vi "FL Convert fc to fs.vi"(8 "error in (no error)":errorcluster, 11 "old controller in":T1) -> (0 "error out":errorcluster, 3 "fuzzy system out":T2 {"user MF interpolating polynomials"."coa_x(y) coeff" format="%.4g"; "user MF interpolating polynomials"."Area(y) coeff" format="%.4g"; "user MF interpolating polynomials"."X(y) coeff" format="%.4g"; "user MF interpolating polynomials"."Y(x) coeff" format="%.4g"; "user MF interpolating polynomials"."Y" format="%.4g"; "user MF interpolating polynomials"."X" format="%.4g"; "defuzzification method" items=["Center of Area", "Modified Center of Area", "Center of Sums", "Center of Maximum", "Mean of Maximum"]; "rules"."consequents"."Var Index" min=0; "rules"."consequents"."Cond" items=["=", "!="]; "rules"."consequents"."MF Index" min=0; "rules"."antecedents"."Var Index" min=0; "rules"."antecedents"."Cond" items=["=", "!="]; "rules"."antecedents"."MF Index" min=0; "rules"."consequent implication" items=["Minimum", "Product"]; "rules"."antecedent connective" items=["AND (Minimum)", "AND (Product)", "OR (Maximum)", "OR (Probabilistic)"]; "output variables"."MFs"."shape" items=["Triangle", "Trapezoid", "Singleton", "Sigmoid", "Gaussian", "User-Defined"]; "input variables"."MFs"."shape" items=["Triangle", "Trapezoid", "Singleton", "Sigmoid", "Gaussian", "User-Defined"]})   [LabVIEW 2017, in "NI_Fuzzy_Logic_API.lvlib"]
uses:
  <vilib>/addons/Fuzzy Logic/NI_Fuzzy_Logic_API.lvlib
  <vilib>/addons/Fuzzy Logic/TypeDefs/FL System.ctl
  <vilib>/addons/Fuzzy Logic/TypeDefs/FL Variable.ctl
  <vilib>/addons/Fuzzy Logic/TypeDefs/FL Membership Function.ctl
  <vilib>/addons/Fuzzy Logic/TypeDefs/FL Membership Function Shape.ctl
  <vilib>/addons/Fuzzy Logic/TypeDefs/FL Rule.ctl
  <vilib>/addons/Fuzzy Logic/TypeDefs/FL Antecedent.ctl
  <vilib>/addons/Fuzzy Logic/TypeDefs/FL Modifier.ctl
  <vilib>/addons/Fuzzy Logic/TypeDefs/FL Antecedent Connective.ctl
  <vilib>/addons/Fuzzy Logic/TypeDefs/FL Consequent.ctl
  <vilib>/addons/Fuzzy Logic/TypeDefs/FL Consequent Implication.ctl
  <vilib>/addons/Fuzzy Logic/TypeDefs/FL Defuzzification.ctl
  <vilib>/addons/Fuzzy Logic/TypeDefs/FL Interpolating polynomials.ctl
  <vilib>/addons/Fuzzy Logic/Membership/FL Create Membership Function (Trapezoid).vi
  <vilib>/Analysis/NI_AALPro.lvlib
panel:
  # "IF"
  # "THEN"
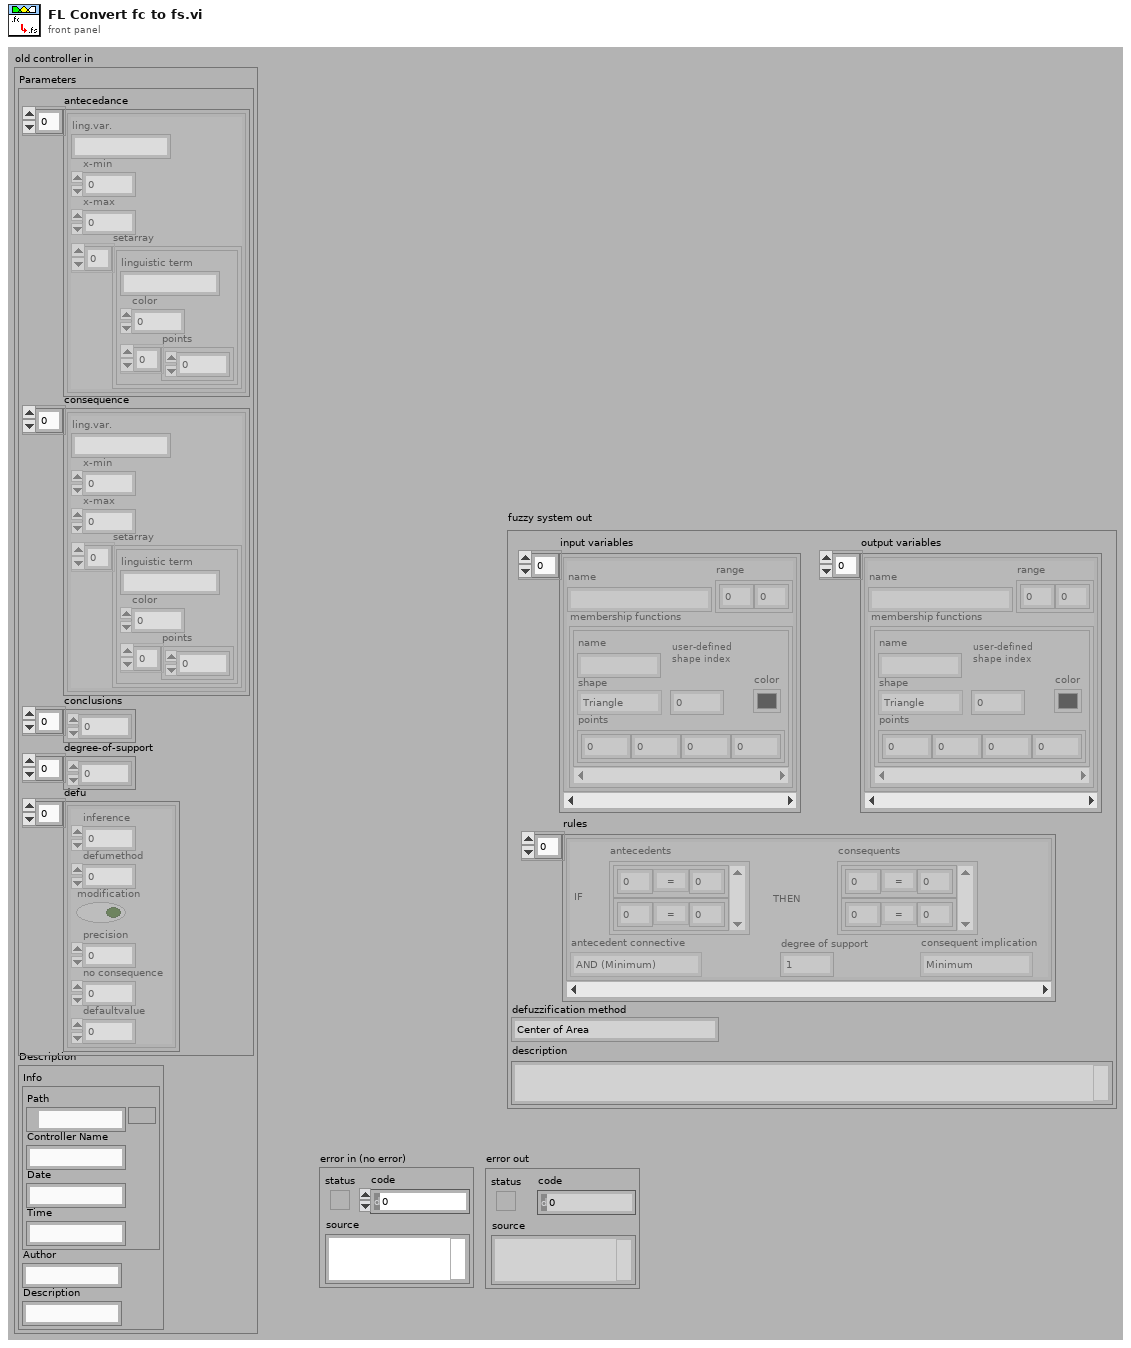
[diagram p1: front panel]
types:
  T1 = cluster{"Parameters":cluster{"antecedance":cluster{"ling.var.":string, "x-min":dbl, "x-max":dbl, "setarray":cluster{"linguistic term":string, "color":u32, "points":dbl[]}[]}[], "consequence":cluster{"ling.var.":string, "x-min":dbl, "x-max":dbl, "setarray":cluster{"linguistic term":string, "color":u32, "points":dbl[]}[]}[], "conclusions":u16[], "degree-of-support":dbl[], "defu":cluster{"inference":u16, "defumethod":u16, "modification":bool, "precision":u16, "no consequence":u16, "defaultvalue":dbl}[]}, "Description":cluster{"Info":cluster{"Path":path, "Controller Name":string, "Date":string, "Time":string}, "Author":string, "Description":string}}
  T2 = typedef "NI_Fuzzy_Logic_API.lvlib/FL System.ctl" = cluster{"input variables":T3[], "output variables":T3[], "rules":T6[], "defuzzification method":T12, "description":string, "user MF interpolating polynomials":T13[]}
  T3 = typedef "NI_Fuzzy_Logic_API.lvlib/FL Variable.ctl" = cluster{"name":string, "range":dbl[], "MFs":T4[]}
  T4 = typedef "NI_Fuzzy_Logic_API.lvlib/FL Membership Function.ctl" = cluster{"name":string, "shape":T5, "points":dbl[], "color":u32, "user-defined shape index":i32}
  T5 = typedef "NI_Fuzzy_Logic_API.lvlib/FL Membership Function Shape.ctl" = u16
  T6 = typedef "NI_Fuzzy_Logic_API.lvlib/FL Rule.ctl" = cluster{"antecedents":T7[], "antecedent connective":T9, "consequents":T10[], "consequent implication":T11, "degree of support":dbl}
  T7 = typedef "NI_Fuzzy_Logic_API.lvlib/FL Antecedent.ctl" = cluster{"Var Index":i32, "MF Index":i32, "Cond":T8}
  T8 = typedef "NI_Fuzzy_Logic_API.lvlib/FL Modifier.ctl" = u16
  T9 = typedef "NI_Fuzzy_Logic_API.lvlib/FL Antecedent Connective.ctl" = u16
  T10 = typedef "NI_Fuzzy_Logic_API.lvlib/FL Consequent.ctl" = cluster{"Var Index":i32, "MF Index":i32, "Cond":T8}
  T11 = typedef "NI_Fuzzy_Logic_API.lvlib/FL Consequent Implication.ctl" = u16
  T12 = typedef "NI_Fuzzy_Logic_API.lvlib/FL Defuzzification.ctl" = u16
  T13 = typedef "NI_Fuzzy_Logic_API.lvlib/FL Interpolating polynomials.ctl" = cluster{"X":dbl[], "Y":dbl[], "Y(x) coeff":dbl[][], "X(y) coeff":dbl[][], "Area(y) coeff":dbl[][], "coa_x(y) coeff":dbl[][]}
  T14 = cluster{"antecedance":cluster{"ling.var.":string, "x-min":dbl, "x-max":dbl, "setarray":cluster{"linguistic term":string, "color":u32, "points":dbl[]}[]}[], "consequence":cluster{"ling.var.":string, "x-min":dbl, "x-max":dbl, "setarray":cluster{"linguistic term":string, "color":u32, "points":dbl[]}[]}[], "conclusions":u16[], "degree-of-support":dbl[], "defu":cluster{"inference":u16, "defumethod":u16, "modification":bool, "precision":u16, "no consequence":u16, "defaultvalue":dbl}[]}
  T15 = cluster{"Info":cluster{"Path":path, "Controller Name":string, "Date":string, "Time":string}, "Author":string, "Description":string}
  T16 = cluster{"ling.var.":string, "x-min":dbl, "x-max":dbl, "setarray":cluster{"linguistic term":string, "color":u32, "points":dbl[]}[]}[]
  T17 = cluster{"inference":u16, "defumethod":u16, "modification":bool, "precision":u16, "no consequence":u16, "defaultvalue":dbl}[]
  T18 = cluster{"linguistic term":string, "color":u32, "points":dbl[]}[]
  T19 = cluster{"inference":u16, "defumethod":u16, "modification":bool, "precision":u16, "no consequence":u16, "defaultvalue":dbl}
  T20 = cluster{"Path":path, "Controller Name":string, "Date":string, "Time":string}
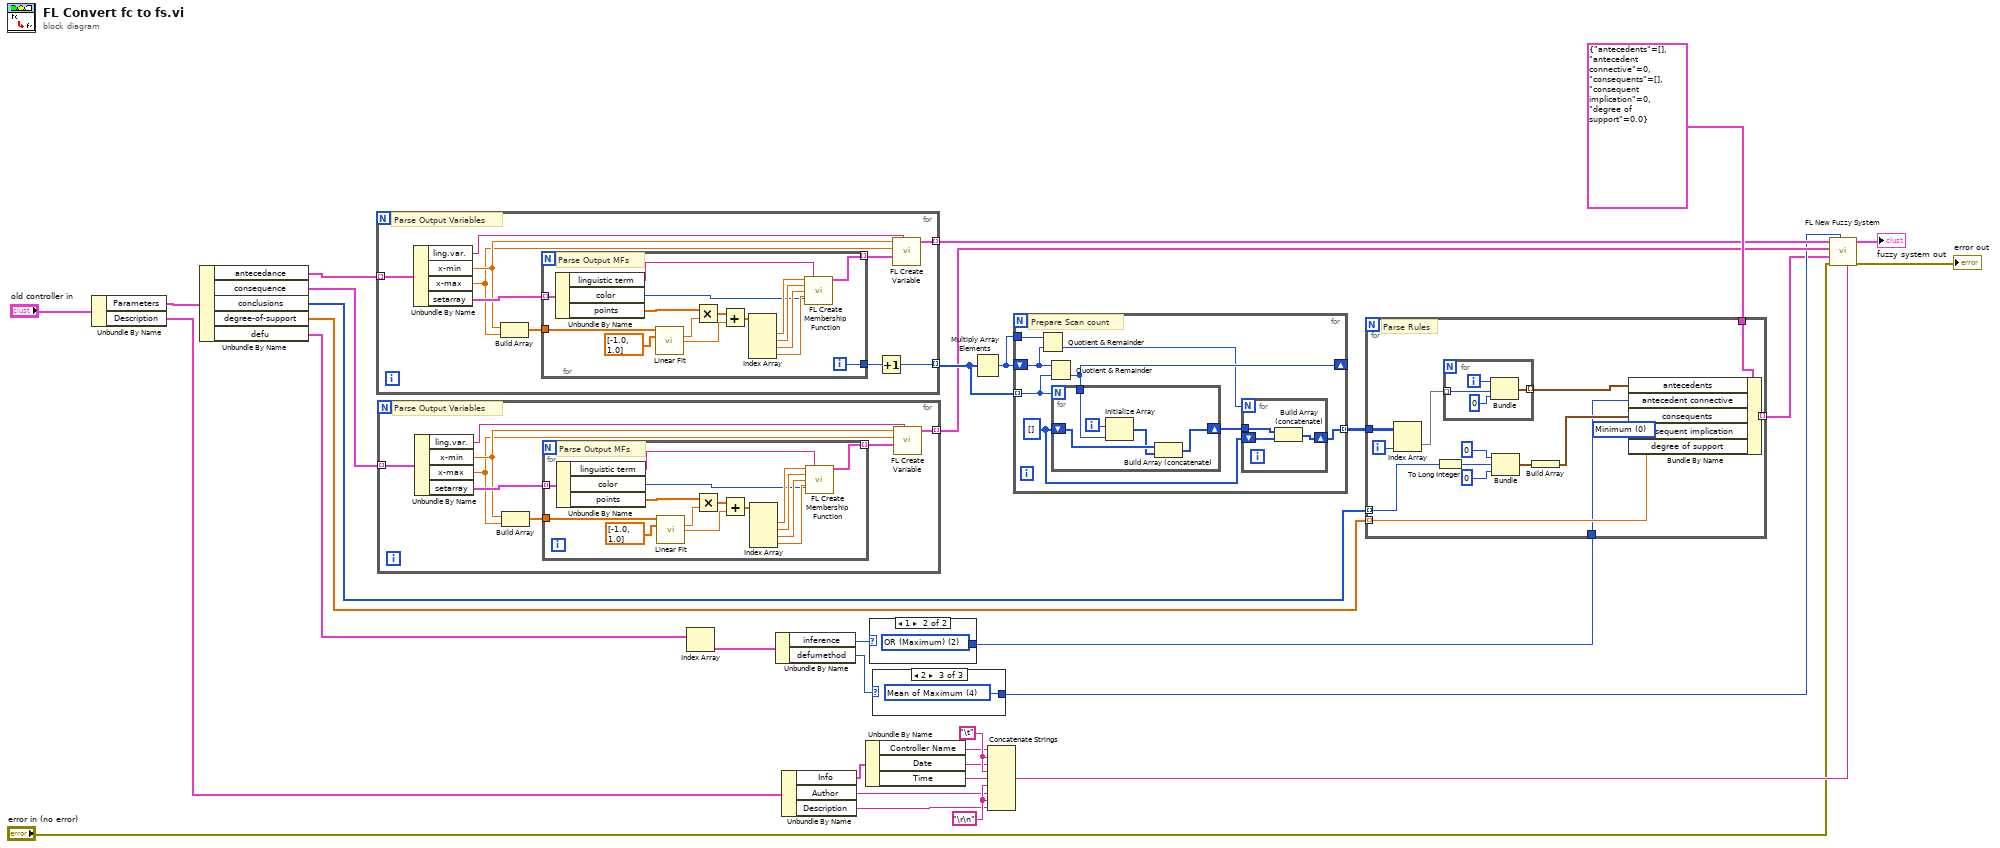
[diagram p0: block diagram]
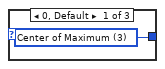
[diagram p2: hidden frame]
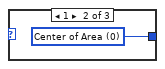
[diagram p3: hidden frame]
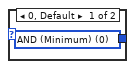
[diagram p4: hidden frame]
diagram:
  w27 = "\t"
  w32 = "\r\n"
  n1 = Unbundle By Name("old controller in") -> ("Parameters"=w12:T14, "Description"=w23:T15)
  n2 = Unbundle By Name(w12) -> ("antecedance"=w10:T16, "consequence"=w13:T16, "conclusions"=w14:u16[], "degree-of-support"=w17:dbl[], "defu"=w18:T17)
  n3 = for {
    tunnel: w10 -> [w42] mode=indexing
    tunnel: [w37] -> w8 mode=indexing
    tunnel: [w33] -> w9 mode=indexing
    # "Parse Output Variables"
    n4 = Unbundle By Name(w42) -> ("ling.var."=w39:string, "x-min"=w36:dbl, "x-max"=w35:dbl, "setarray"=w41:T18)
    n5 = Build Array(w36, w35) -> (w40:dbl[])
    n6 = for {
      tunnel: w41 -> [w58] mode=indexing
      tunnel: w40 -> [w53]
      tunnel: [w45] -> w38 mode=indexing
      tunnel: [w43] -> w34
      i -> [w43]
      # "Parse Output MFs"
      n7 = Unbundle By Name(w58) -> ("linguistic term"=w44:string, "color"=w46:u32, "points"=w52:dbl[])
      n8 = call <vilib>:"Linear Fit.vi"("Y"=w53, "X"=dbl[] [-1.0, 1.0] ("Y")) -> ("slope"=w57:dbl, "intercept"=w56:dbl)  [unwired: 4 in, 8 out]
      n9 = Multiply(x=w52, y=w57) -> (x*y=w55:dbl[])
      n10 = Add(x=w55, y=w56) -> (x+y=w51:dbl[])
      n11 = Index Array(array=w51) -> (element #1=w50:dbl, element #2=w49:dbl, element #3=w48:dbl, element #4=w47:dbl)  [unwired: 4 in]
      n12 = call-poly <vilib>:"FL Create Membership Function.vi"("left base"=w50, "name"=w44, "left top"=w49, "right top"=w48, "right base"=w47, "color"=w46) -> ("membership function"=w45:T4)  [unwired: 1 in, 8 out]
    }
    n13 = Increment(x=w34) -> (x+1=w33:i32)
    n14 = call <vilib>:"FL Create Variable.vi"("name"=w39, "membership functions"=w38, "maximum"=w35, "minimum"=w36) -> ("variable"=w37:T3)  [unwired: 1 in, 6 out]
  }
  n15 = for {
    tunnel: w13 -> [w66] mode=indexing
    tunnel: [w61] -> w7 mode=indexing
    # "Parse Output Variables"
    n16 = Unbundle By Name(w66) -> ("ling.var."=w63:string, "x-min"=w60:dbl, "x-max"=w59:dbl, "setarray"=w65:T18)
    n17 = Build Array(w60, w59) -> (w64:dbl[])
    n18 = for {
      tunnel: w65 -> [w81] mode=indexing
      tunnel: w64 -> [w76]
      tunnel: [w68] -> w62 mode=indexing
      # "Parse Output MFs"
      n19 = Unbundle By Name(w81) -> ("linguistic term"=w67:string, "color"=w69:u32, "points"=w75:dbl[])
      n20 = call <vilib>:"Linear Fit.vi"("Y"=w76, "X"=dbl[] [-1.0, 1.0] ("Y")) -> ("slope"=w80:dbl, "intercept"=w79:dbl)  [unwired: 4 in, 8 out]
      n21 = Multiply(x=w75, y=w80) -> (x*y=w78:dbl[])
      n22 = Add(x=w78, y=w79) -> (x+y=w74:dbl[])
      n23 = Index Array(array=w74) -> (element #1=w73:dbl, element #2=w72:dbl, element #3=w71:dbl, element #4=w70:dbl)  [unwired: 4 in]
      n24 = call-poly <vilib>:"FL Create Membership Function.vi"("left base"=w73, "name"=w67, "left top"=w72, "right top"=w71, "right base"=w70, "color"=w69) -> ("membership function"=w68:T4)  [unwired: 1 in, 8 out]
    }
    n25 = call <vilib>:"FL Create Variable.vi"("name"=w63, "membership functions"=w62, "maximum"=w59, "minimum"=w60) -> ("variable"=w61:T3)  [unwired: 1 in, 6 out]
  }
  n26 = Index Array(array=w18) -> (element=w19:T19)  [unwired: 1 in]
  n27 = Unbundle By Name(w19) -> ("inference"=w20:u16, "defumethod"=w21:u16)
  n28 = Unbundle By Name(w23) -> ("Info"=w24:T20, "Author"=w29:string, "Description"=w30:string)
  n29 = Unbundle By Name(w24) -> ("Controller Name"=w25:string, "Date"=w26:string, "Time"=w28:string)
  n30 = case shown="1" w20 {
    tunnel: [w82 w83] -> w22
    frame 0, Default {
      w82 = T9 0 items=["AND (Minimum)", "AND (Product)", "OR (Maximum)", "OR (Probabilistic)"] ("Operation")
    }
    frame 1 {
      w83 = T9 2 items=["AND (Minimum)", "AND (Product)", "OR (Maximum)", "OR (Probabilistic)"] ("Operation")
    }
  }
  n31 = case shown="2" w21 {
    tunnel: [w84 w85 w86] -> w6
    frame 0, Default {
      w84 = T12 3 items=["Center of Area", "Modified Center of Area", "Center of Sums", "Center of Maximum", "Mean of Maximum"] ("Defuzzification")
    }
    frame 1 {
      w85 = T12 0 items=["Center of Area", "Modified Center of Area", "Center of Sums", "Center of Maximum", "Mean of Maximum"] ("Defuzzification")
    }
    frame 2 {
      w86 = T12 4 items=["Center of Area", "Modified Center of Area", "Center of Sums", "Center of Maximum", "Mean of Maximum"] ("Defuzzification")
    }
  }
  n32 = Multiply Array Elements(1:w9) -> (0:w15:i32)
  n33 = Concatenate Strings(w25, w27, w26, w27, w28, w32, w29, w32, w30) -> (w5:string)
  n34 = for {
    tunnel: w9 -> [w94] mode=indexing
    tunnel: [w91] -> w16 mode=indexing
    shift-right: [w93] -> _
    shift-left: w15 -> [w89]
    tunnel: w15 -> [w90]
    w87 = i32[] []
    # "Prepare Scan count"
    n35 = Quotient & Remainder(x=w90, y=w89) -> (floor(x/y)=w88:i32)  [unwired: 1 out]
    n36 = Quotient & Remainder(x=w89, y=w94) -> (floor(x/y)=w93:i32)  [unwired: 1 out]
    n37 = for {
      N: w94 -> [_]
      tunnel: w93 -> [w101]
      shift-right: [w98] -> w92
      shift-left: w87 -> [w100]
      i -> [w102]
      n38 = Initialize Array(w102, w101) -> (w99:i32[])
      n39 = Build Array (concatenate)(w100, w99) -> (w98:i32[])
    }
    n40 = for {
      N: w88 -> [_]
      shift-right: [w95] -> w91
      shift-left: w87 -> [w97]
      tunnel: w92 -> [w96]
      n41 = Build Array (concatenate)(w96, w97) -> (w95:i32[])
    }
  }
  n42 = for {
    tunnel: [w117] -> w4 mode=indexing
    tunnel: w14 -> [w113] mode=indexing
    tunnel: w16 -> [w116]
    tunnel: w17 -> [w105] mode=indexing
    tunnel: w22 -> [w104]
    tunnel: T6 {"antecedents"=[], "antecedent connective"=0, "consequents"=[], "consequent implication"=0, "degree of support"=0.0} ("Rule") -> [w108]
    i -> [w115]
    w103 = T11 0 items=["Minimum", "Product"] ("Implication")
    # "Parse Rules"
    n43 = Index Array(array=w116, index (col)=w115) -> (element=w114:i32[])  [unwired: 1 in]
    n44 = To Long Integer(number=w113) -> (32bit integer=w112:i32)
    n45 = for {
      tunnel: w114 -> [w120] mode=indexing
      tunnel: [w119] -> w107 mode=indexing
      i -> [w121]
      n46 = Bundle(w121, w120, "Cond"=u16 0) -> (w119:cluster{i32, i32, "Cond":u16})  [unwired: 1 out]
    }
    n47 = Bundle("32bit integer"=0, w112, "Cond"=u16 0) -> (w110:cluster{"32bit integer":i32, i32, "Cond":u16})  [unwired: 1 out]
    n48 = Build Array(w110) -> (w106:cluster{"32bit integer":i32, i32, "Cond":u16}[])
    n49 = Bundle By Name(cluster=w108, "antecedents"=w107, "antecedent connective"=w104, "consequents"=w106, "consequent implication"=w103, "degree of support"=w105) -> (w117:T6)
  }
  n50 = call <vilib>:"FL New Fuzzy System.vi"("description"=w5, "defuzzification method"=w6, "error in (no error)"="error in (no error)", "rules"=w4, "output variables"=w7, "input variables"=w8) -> ("error out"=→"error out":errorcluster, "fuzzy system out"=→"fuzzy system out":T2)  [unwired: 1 in, 3 out]
